vi "MD5 FGHI functions__ogtk.vi"(4 "ti":u32, 6 "s":i32, 7 "Mj":u32, 9 "Operator function":enum16{"F", "G", "H", "I"}(ring), 11 "Chaining Variables":u32[](array[numeric])) -> (3 "Resulting Chaining Variables":u32[](array[numeric]))   [LabVIEW 2009]
panel:
  # "[OpenG VI Tags] ***Do Not Remove***"
  # "MD5 FGHI.vi\n\nDerived from the RSA Data Security, Inc. MD5 Message-Digest Algorithm\n\nPlease visit http://www.OpenG.org to learn about the\nOpen Source LabVIEW software movement.\n\nNOTICE -- YOU MUST LEAVE THIS NOTICE IN PLACE.  PER THE TERMS OF THE LICENSE BELOW, YOU MAY SUBLICENSE THIS SOFTWARE \nIN ANY WAY THAT DOES NOT CONFLICT WITH THIS LICENSE.\n\n### BSD License (http://www.opensource.org/licenses/bsd-license.php) Begin ###\n \nCopyright (c) 2004, Enrique Vargas <vargas@visecurity.com>\n\nAll rights reserved.\n\nRedistribution and use in source and binary forms, with or without modification, are permitted provided that the following conditions are met:\n\n    * Redistributions of source code must retain the above copyright notice, this list of conditions and the following disclaimer.\n    * Redistributions in binary form must reproduce the above copyright notice, this list of conditions and the following disclaimer in the \n       documentation and/or other materials provided with the distribution.\n    * Neither the name of SciWare, James Kring, Inc., nor the names of its contributors may be used to endorse or promote products derived \n       from this software without specific prior written permission.\n\nTHIS SOFTWARE IS PROVIDED BY THE COPYRIGHT HOLDERS AND CONTRIBUTORS \"AS IS\" AND ANY EXPRESS OR IMPLIED WARRANTIES, \nINCLUDING, BUT NOT LIMITED TO, THE IMPLIED WARRANTIES OF MERCHANTABILITY AND FITNESS FOR A PARTICULAR PURPOSE ARE \nDISCLAIMED. IN NO EVENT SHALL THE COPYRIGHT OWNER OR CONTRIBUTORS BE LIABLE FOR ANY DIRECT, INDIRECT, INCIDENTAL,\n SPECIAL, EXEMPLARY, OR CONSEQUENTIAL DAMAGES (INCLUDING, BUT NOT LIMITED TO, PROCUREMENT OF SUBSTITUTE GOODS OR \nSERVICES; LOSS OF USE, DATA, OR PROFITS; OR BUSINESS INTERRUPTION) HOWEVER CAUSED AND ON ANY THEORY OF LIABILITY, \nWHETHER IN CONTRACT, STRICT LIABILITY, OR TORT (INCLUDING NEGLIGENCE OR OTHERWISE) ARISING IN ANY WAY OUT OF THE USE \nOF THIS SOFTWARE, EVEN IF ADVISED OF THE POSSIBILITY OF SUCH DAMAGE.\n\n### BSD License End ###"
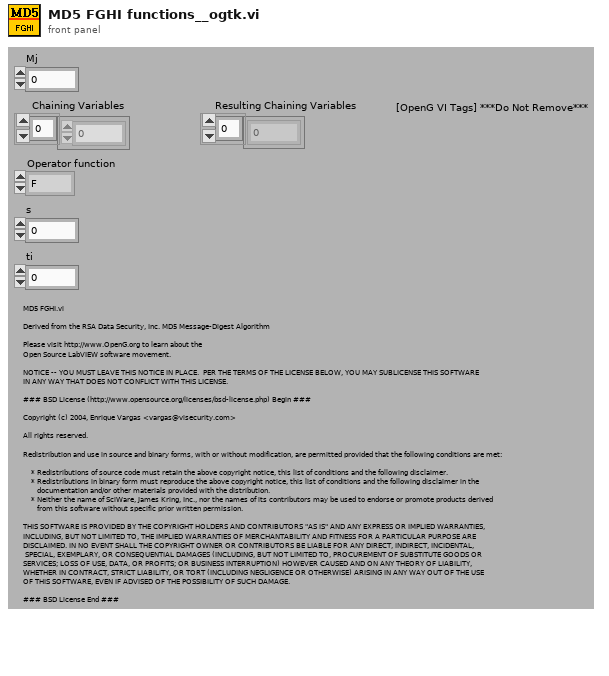
[diagram p1: front panel]
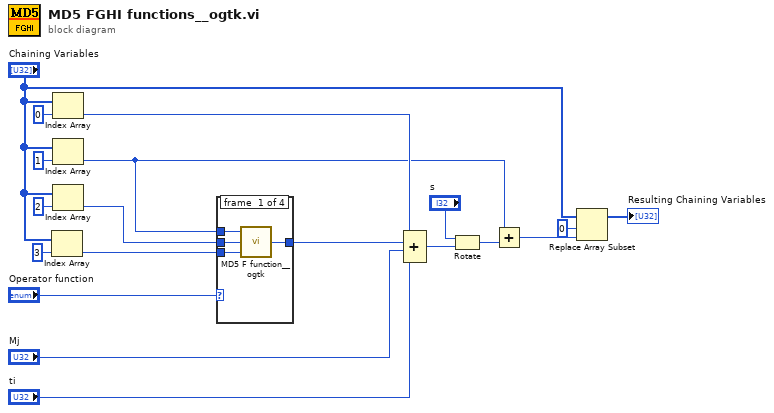
[diagram p0: block diagram]
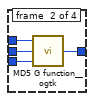
[diagram p2: hidden frame]
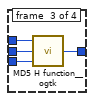
[diagram p3: hidden frame]
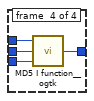
[diagram p4: hidden frame]
diagram:
  n1 = Index Array(array="Chaining Variables", index=3 ("Index")) -> (element=w7:u32)
  n2 = Index Array(array="Chaining Variables", index=0 ("Index")) -> (element=w10:u32)
  n3 = Index Array(array="Chaining Variables", index=1 ("Index")) -> (element=w9:u32)
  n4 = Index Array(array="Chaining Variables", index=2 ("Index")) -> (element=w8:u32)
  n5 = case shown="\"G\"" "Operator function" {
    tunnel: [w23 w24 w28 w32] -> w19
    tunnel: w9 -> [w22 w26 w30 w34]
    tunnel: w8 -> [w21 w25 w29 w33]
    tunnel: w7 -> [w20 w27 w31 w35]
    frame #0 {
      n6 = call "MD5 F function__ogtk.vi"("Z"=w20, "Y"=w21, "X"=w22) -> ("F(X,Y,Z)"=w23:u32)
    }
    frame #1 {
      n7 = call "MD5 G function__ogtk.vi"("Z"=w27, "Y"=w25, "X"=w26) -> ("G(X,Y,Z)"=w24:u32)
    }
    frame #2 {
      n8 = call "MD5 H function__ogtk.vi"("Z"=w31, "Y"=w29, "X"=w30) -> ("H(X,Y,Z)"=w28:u32)
    }
    frame #3 {
      n9 = call "MD5 I function__ogtk.vi"("Z"=w35, "Y"=w33, "X"=w34) -> ("I(X,Y,Z)"=w32:u32)
    }
  }
  n10 = Compound Arithmetic op=ADD(w10, w19, "Mj", "ti") -> (w16:u32)
  n11 = Rotate(1:w16, 2:"s") -> (0:w15:u32)
  n12 = Add(x=w9, y=w15) -> (x+y=w6:u32)
  n13 = Replace Array Subset(array="Chaining Variables", new element=w6, index=0 ("Index")) -> (→"Resulting Chaining Variables":u32[])
